vi "AIT 664 - Read XML Configuration File.vi"(0 "Path":path, 11 "error in (no error)":errorcluster) -> (4 "Path out":path, 6 "664 Device":T1, 15 "error out":errorcluster)   [LabVIEW 2013, in "AIT 664 Custom Device.lvlib"]
doc: "Parse the xml configuration file."
uses:
  AIT 664 Custom Device.lvlib
  Controls/664 - XML Device Description.ctl
  Controls/664 - XML End System Description.ctl
  Controls/664 - XML Output VL.ctl
  Controls/664 - XML Tx Message Port.ctl
  Controls/664 - Sampling Type.ctl
  Controls/664 -Param.ctl
  Controls/664 - XML Input VL.ctl
  Controls/664 - XML Rx Message Port.ctl
  <vilib>/xml/Load XML File.vi
  <vilib>/xml/Close Reference(Node).vi
  <vilib>/xml/NI_XML.lvlib
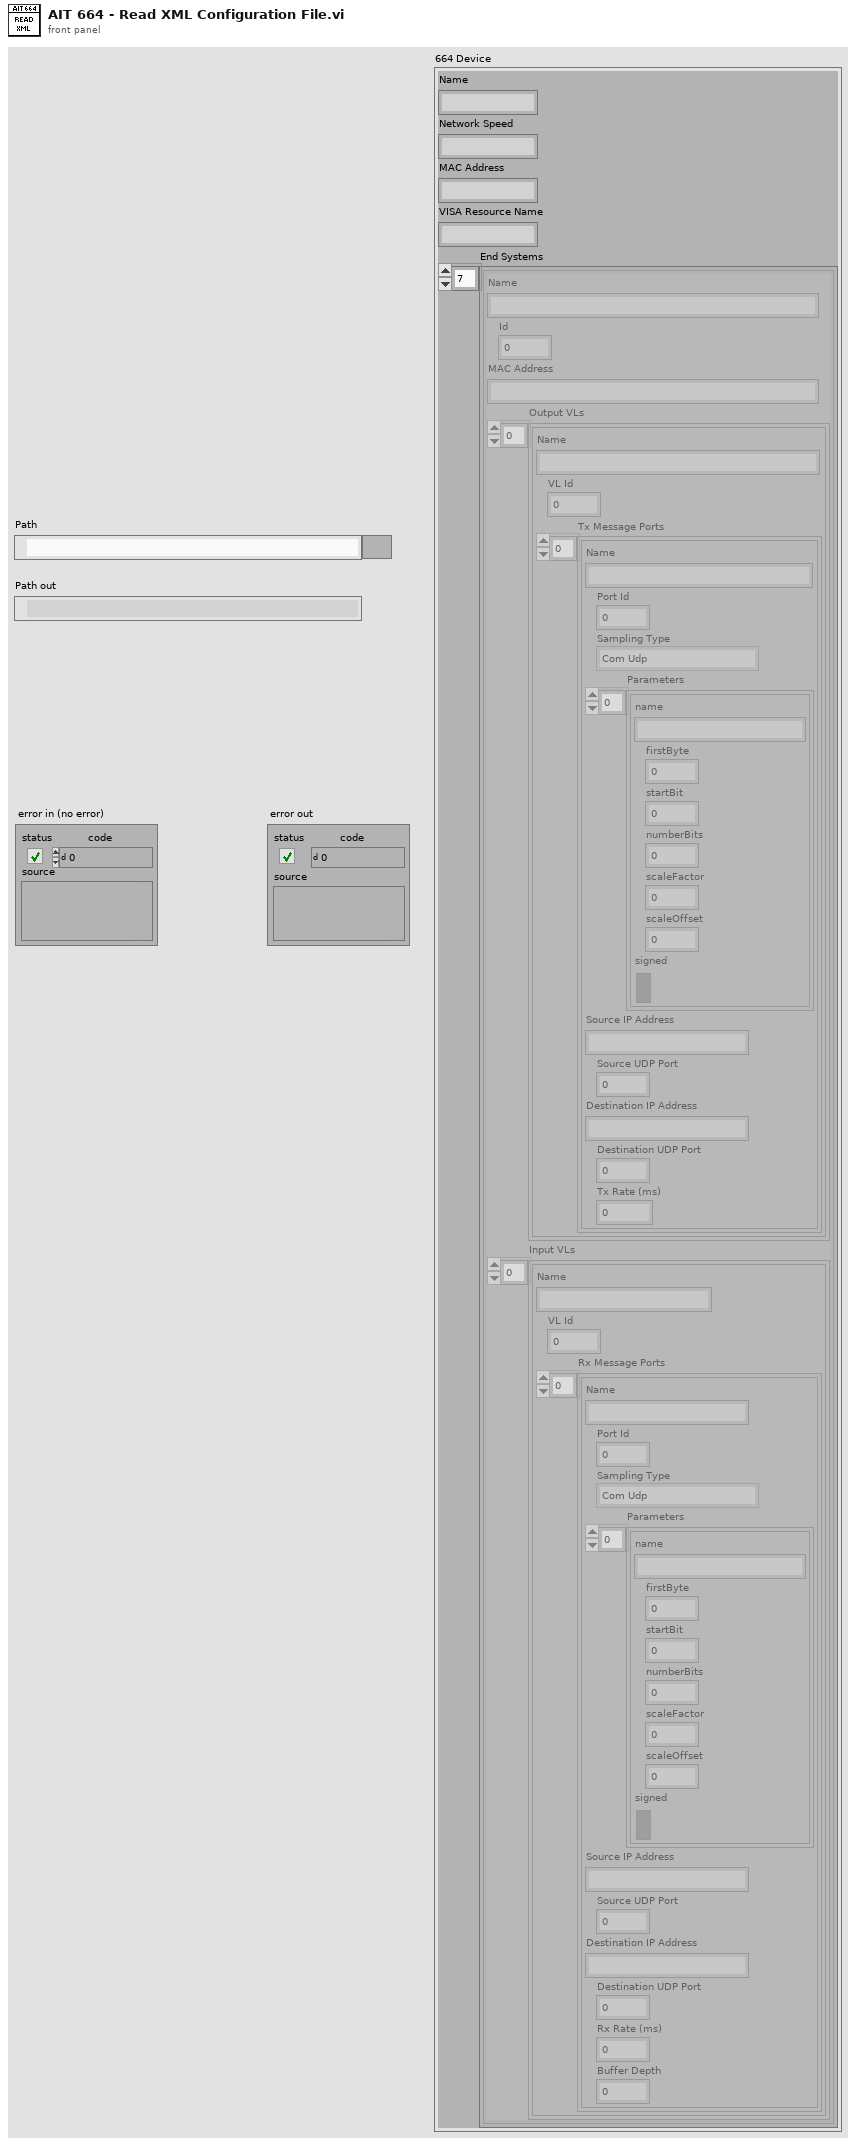
[diagram p1: front panel]
types:
  T1 = typedef "AIT 664 Custom Device.lvlib/664 - XML Device Description.ctl" = cluster{"Name":string, "Network Speed":string, "MAC Address":string, "VISA Resource Name":string, "End Systems":T2[]}
  T2 = typedef "AIT 664 Custom Device.lvlib/664 - XML End System Description.ctl" = cluster{"Name":string, "Id":u32, "MAC Address":string, "Output VLs":T3[], "Input VLs":T7[]}
  T3 = typedef "AIT 664 Custom Device.lvlib/664 - XML Output VL.ctl" = cluster{"Name":string, "VL Id":u32, "Tx Message Ports":T4[]}
  T4 = typedef "AIT 664 Custom Device.lvlib/664 - XML Tx Message Port.ctl" = cluster{"Name":string, "Port Id":u32, "Sampling Type":T5, "Parameters":T6[], "Source IP Address":string, "Source UDP Port":u32, "Destination IP Address":string, "Destination UDP Port":u32, "Tx Rate (ms)":u32}
  T5 = typedef "AIT 664 Custom Device.lvlib/664 - Sampling Type.ctl" = enum16{"Com Udp", "Com Udp Queuing", "Sap Udp", "Sap Ip", "Sap Mac", "Unknown"}
  T6 = typedef "AIT 664 Custom Device.lvlib/664 -Param.ctl" = cluster{"name":string, "firstByte":i32, "startBit":i32, "numberBits":i32, "scaleFactor":dbl, "scaleOffset":dbl, "signed":bool}
  T7 = typedef "AIT 664 Custom Device.lvlib/664 - XML Input VL.ctl" = cluster{"Name":string, "VL Id":u32, "Rx Message Ports":T8[]}
  T8 = typedef "AIT 664 Custom Device.lvlib/664 - XML Rx Message Port.ctl" = cluster{"Name":string, "Port Id":u32, "Sampling Type":T5, "Parameters":T6[], "Source IP Address":string, "Source UDP Port":u32, "Destination IP Address":string, "Destination UDP Port":u32, "Rx Rate (ms)":u32, "Buffer Depth":u32}
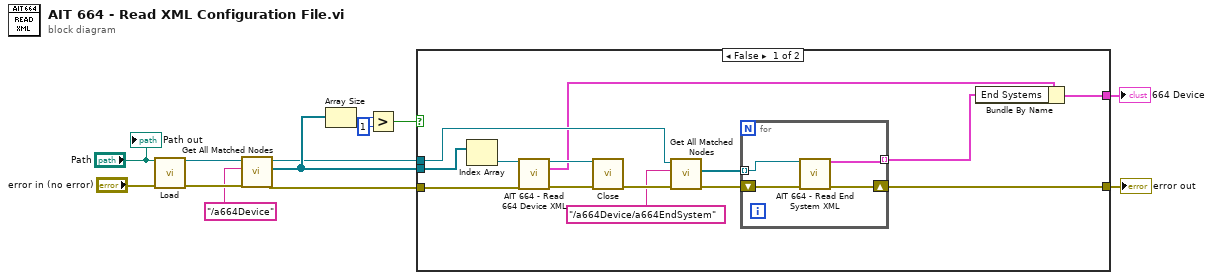
[diagram p0: block diagram]
diagram:
  n1 = call-poly <vilib>:"Load.vi"("path to XML document"="Path", "error in (no error)"="error in (no error)") -> ("DOM document out"=w10:refnum<k20>, "error out"=w12:errorcluster)  [unwired: 11 in, 1 out]
  n2 = call <vilib>:"Get All Matched Nodes.vi"("error in (no error)"=w12, "XPath expression"="/a664Device", "node in"=w10) -> ("error out"=w5:errorcluster, "node result array"=w6:refnum<k20>[], "node out"=w3:refnum<k20>)  [unwired: 6 out]
  n3 = Array Size(array=w6) -> (size(s)=w9:i32)
  n4 = Greater?(x=w9, y=1) -> (0:w7:bool)
  n5 = case shown="False" w7 {
    tunnel: w6 -> [w27 _]
    tunnel: w5 -> [w26 w32]
    tunnel: w3 -> [w21 _]
    tunnel: [w17 w32] -> w1
    tunnel: [w14 _] -> w2
    frame False {
      n6 = Index Array(array=w27) -> (element=w25:refnum<k20>)  [unwired: 1 in]
      n7 = call "AIT 664 - Read 664 Device XML.vi"("Refnum in"=w25, "error in (no error)"=w26) -> ("Refnum out"=w23:refnum<k20>, "664 Device"=w16:T1, "error out"=w24:errorcluster)  [unwired: 11 in]
      n8 = call-poly <vilib>:"Close.vi"("error in (no error)"=w24, "node"=w23) -> ("error out"=w22:errorcluster)  [unwired: 7 in]
      n9 = call <vilib>:"Get All Matched Nodes.vi"("error in (no error)"=w22, "XPath expression"="/a664Device/a664EndSystem", "node in"=w21) -> ("error out"=w18:errorcluster, "node result array"=w19:refnum<k20>[])  [unwired: 7 out]
      n10 = for {
        tunnel: w19 -> [w30] mode=indexing
        tunnel: [w28] -> w15 mode=indexing
        shift-right: [w29] -> w17
        shift-left: w18 -> [w31]
        n11 = call "AIT 664 - Read End System XML.vi"("Refnum in"=w30, "error in (no error)"=w31) -> ("664 End System"=w28:T2, "error out"=w29:errorcluster)  [unwired: 12 in]
      }
      n12 = Bundle By Name(cluster=w16, "End Systems"=w15) -> (w14:T1)
    }
    frame True {
      # "xxx Report error, only one 664 device per xml file"
    }
  }
  "664 Device" <- w2
  "error out" <- w1
  "Path out" <- "Path"
